vi "make_value_pairs.vi"(7 "Value Pair Properties":T6={"X Value Pairs"={"Data Array"=[], "Show ticks"=TRUE, "Show grid lines"=TRUE, "Labels"=enum."Name"}, "Y Value Pairs"={"Data Array"=[], "Show ticks"=TRUE, "Show grid lines"=TRUE, "Labels"=enum."Value"}, "Z Value Pairs"={"Data Array"=[], "Show ticks"=TRUE, "Show grid lines"=TRUE, "Labels"=enum."Value"}}, 9 "Format strings":T1, 10 "Ticks Properties.Major Count":cluster{"X":i32, "Y":i32, "Z":i32}, 11 "Range Min/Max":T4) -> (3 "Axis output cluster":T2)   [LabVIEW 2020, in "3DPC_SurfacePlot.xctl"]
uses:
  <vilib>/Native 3D Graph/xcontrol/3DPC_SurfacePlot.xctl
  <vilib>/Native 3D Graph/typedefs/prop_value_pair_all.ctl
  <vilib>/Native 3D Graph/typedefs/prop_value_pair_1d.ctl
  <vilib>/Native 3D Graph/typedefs/range_cluster.ctl
  <vilib>/Native 3D Graph/typedefs/min_max.ctl
  <vilib>/Native 3D Graph/typedefs/prop_axes_merged_array_etc.ctl
  <vilib>/Native 3D Graph/typedefs/prop_axes_merged_array.ctl
  <vilib>/Native 3D Graph/typedefs/prop_format.ctl
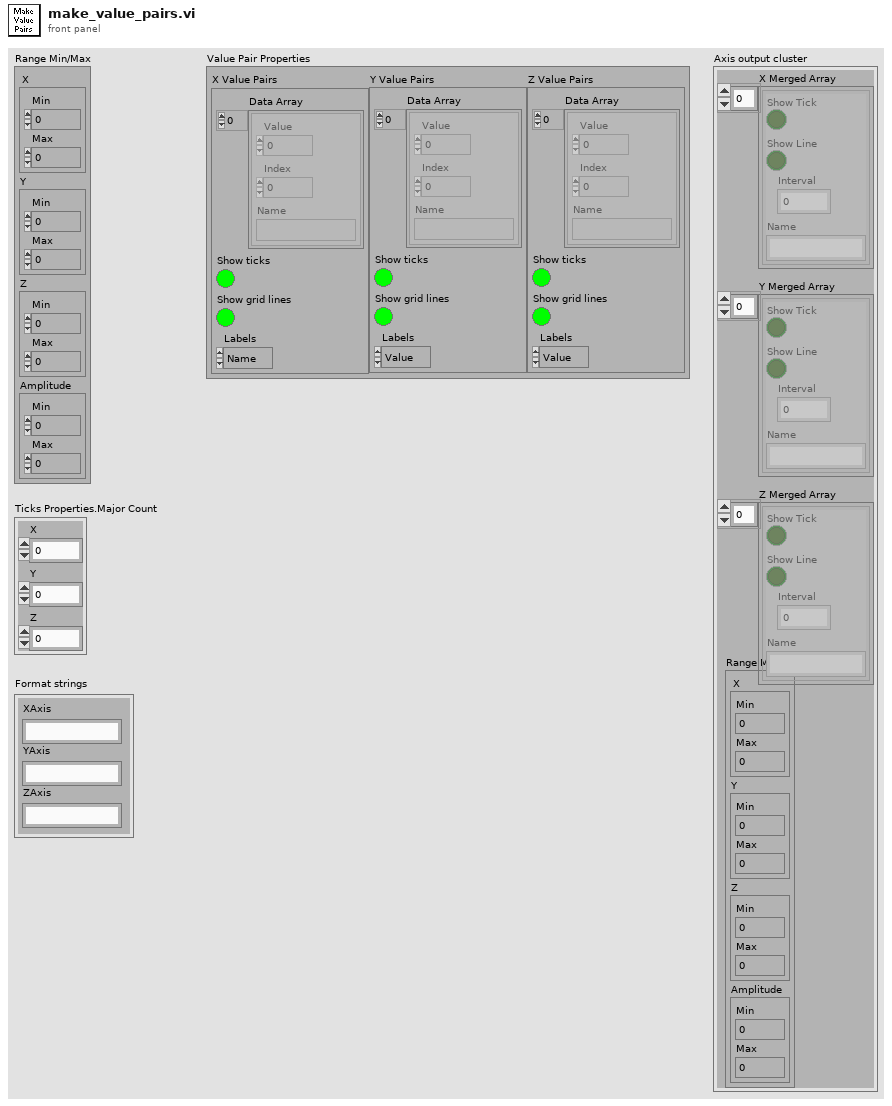
[diagram p1: front panel]
types:
  T1 = typedef "3DPC_SurfacePlot.xctl/prop_format.ctl" = cluster{"XAxis":string, "YAxis":string, "ZAxis":string}
  T2 = typedef "3DPC_SurfacePlot.xctl/prop_axes_merged_array_etc.ctl" = cluster{"X Merged Array":T3, "Y Merged Array":T3, "Z Merged Array":T3, "Range Min/Max":T4}
  T3 = typedef "3DPC_SurfacePlot.xctl/prop_axes_merged_array.ctl" = cluster{"Show Tick":bool, "Show Line":bool, "Interval":sgl, "Name":string}[]
  T4 = typedef "3DPC_SurfacePlot.xctl/range_cluster.ctl" = cluster{"X":T5, "Y":T5, "Z":T5, "Amplitude":T5}
  T5 = typedef "3DPC_SurfacePlot.xctl/min_max.ctl" = cluster{"Min":sgl, "Max":sgl}
  T6 = typedef "3DPC_SurfacePlot.xctl/prop_value_pair_all.ctl" = cluster{"X Value Pairs":cluster{"Data Array":cluster{"Value":sgl, "Index":i32, "Name":string}[], "Show ticks":bool, "Show grid lines":bool, "Labels":enum16{"Value", "None", "Name"}}, "Y Value Pairs":T7, "Z Value Pairs":T7}
  T7 = typedef "3DPC_SurfacePlot.xctl/prop_value_pair_1d.ctl" = cluster{"Data Array":cluster{"Value":sgl, "Index":i32, "Name":string}[], "Show ticks":bool, "Show grid lines":bool, "Labels":enum16{"Value", "None", "Name"}}
  T8 = cluster{"Data Array":cluster{"Value":sgl, "Index":i32, "Name":string}[], "Show ticks":bool, "Show grid lines":bool, "Labels":enum16{"Value", "None", "Name"}}
  T9 = cluster{"Show Tick":bool, "Show Line":bool, "Interval":sgl, "Name":string}[]
  T10 = cluster{"Merged Array Out":cluster{"Show Tick":bool, "Show Line":bool, "Interval":sgl, "Name":string}[], "Merged Array Out":cluster{"Show Tick":bool, "Show Line":bool, "Interval":sgl, "Name":string}[], "Merged Array Out":cluster{"Show Tick":bool, "Show Line":bool, "Interval":sgl, "Name":string}[], "Range Min/Max":T4}
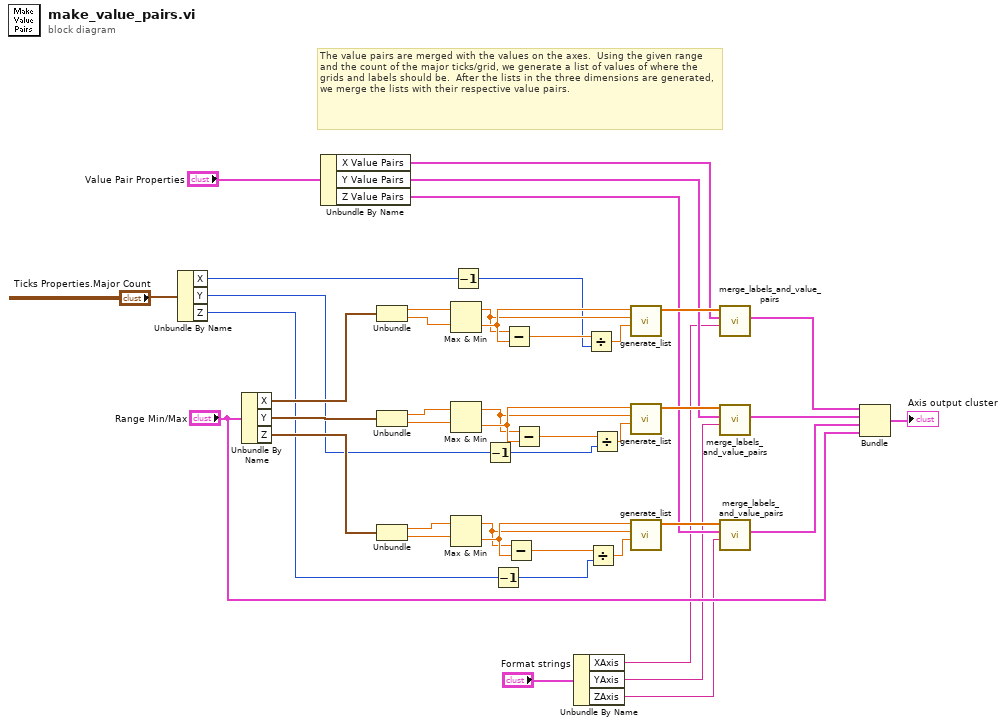
[diagram p0: block diagram]
diagram:
  # "The value pairs are merged with the values on the axes.  Using the given range and the count of the major ticks/grid, we generate a list of values of where the grids and labels should be.  After the lists in the three dimensions are generated, we merge the lists with their respective value pairs."
  n1 = Unbundle By Name("Ticks Properties.Major Count") -> ("X"=w7:i32, "Y"=w6:i32, "Z"=w5:i32)
  n2 = Unbundle By Name("Range Min/Max") -> ("X"=w41:T5, "Y"=w40:T5, "Z"=w39:T5)
  n3 = Unbundle By Name("Value Pair Properties") -> ("X Value Pairs"=w25:T8, "Y Value Pairs"=w24:T7, "Z Value Pairs"=w23:T7)
  n4 = Unbundle(w41) -> ("Min"=w38:sgl, "Max"=w37:sgl)
  n5 = Unbundle(w40) -> ("Min"=w32:sgl, "Max"=w31:sgl)
  n6 = Unbundle(w39) -> ("Min"=w30:sgl, "Max"=w29:sgl)
  n7 = Max & Min(x=w38, y=w37) -> (max(x,y)=w21:sgl, min(x,y)=w22:sgl)
  n8 = Max & Min(x=w32, y=w31) -> (max(x,y)=w19:sgl, min(x,y)=w20:sgl)
  n9 = Max & Min(x=w30, y=w29) -> (max(x,y)=w17:sgl, min(x,y)=w18:sgl)
  n10 = Decrement(x=w7) -> (x-1=w14:i32)
  n11 = Decrement(x=w6) -> (x-1=w15:i32)
  n12 = Decrement(x=w5) -> (x-1=w16:i32)
  n13 = Subtract(x=w21, y=w22) -> (x-y=w43:sgl)
  n14 = Subtract(x=w17, y=w18) -> (x-y=w34:sgl)
  n15 = Subtract(x=w19, y=w20) -> (x-y=w36:sgl)
  n16 = Unbundle By Name("Format strings") -> ("XAxis"=w3:string, "YAxis"=w2:string, "ZAxis"=w1:string)
  n17 = Divide(x=w43, y=w14) -> (x/y=w42:sgl)
  n18 = Divide(x=w34, y=w16) -> (x/y=w33:sgl)
  n19 = Divide(x=w36, y=w15) -> (x/y=w35:sgl)
  n20 = call <vilib>:"generate_list.vi"("Interval"=w42, "End"=w21, "Start"=w22) -> ("Array"=w26:sgl[])  [unwired: 8 out]
  n21 = call <vilib>:"generate_list.vi"("Interval"=w35, "End"=w19, "Start"=w20) -> ("Array"=w27:sgl[])  [unwired: 8 out]
  n22 = call <vilib>:"generate_list.vi"("Interval"=w33, "End"=w17, "Start"=w18) -> ("Array"=w28:sgl[])  [unwired: 8 out]
  n23 = call <vilib>:"merge_labels_and_value_pairs.vi"("Format string"=w3, "Value Pairs"=w25, "Data Array"=w26) -> ("Merged Array Out"=w11:T9)  [unwired: 8 out]
  n24 = call <vilib>:"merge_labels_and_value_pairs.vi"("Format string"=w2, "Value Pairs"=w24, "Data Array"=w27) -> ("Merged Array Out"=w13:T9)  [unwired: 8 out]
  n25 = call <vilib>:"merge_labels_and_value_pairs.vi"("Format string"=w1, "Value Pairs"=w23, "Data Array"=w28) -> ("Merged Array Out"=w12:T9)  [unwired: 8 out]
  n26 = Bundle("Merged Array Out"=w11, "Merged Array Out"=w13, "Merged Array Out"=w12, "Range Min/Max"="Range Min/Max") -> (→"Axis output cluster":T10)  [unwired: 1 out]
